vi "FdxCmdRxSAPReadCvi.vi"(8 "error in":errorcluster, 9 "SapReadIn":cluster{"UdpHandle":u32, "MsgCount":u32}, 11 "InstrumentHandle_port":u32) -> (0 "error out":errorcluster, 1 "SapReadOut":cluster{"MsgRead":u32, "ReadBuffer":u8[]}, 3 "InstrumentHandle_port":u32)   [LabVIEW 2020, in "AIM664LV.lvlib"]
doc: "This function reads data from an SAP Connectionless port."
uses:
  AIM664LV.lvlib
  AFDX_LibraryAdmin/FdxGlobalDllPath.vi
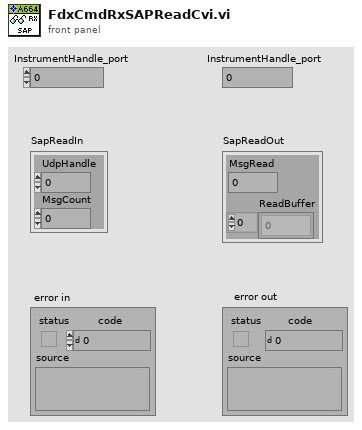
[diagram p1: front panel]
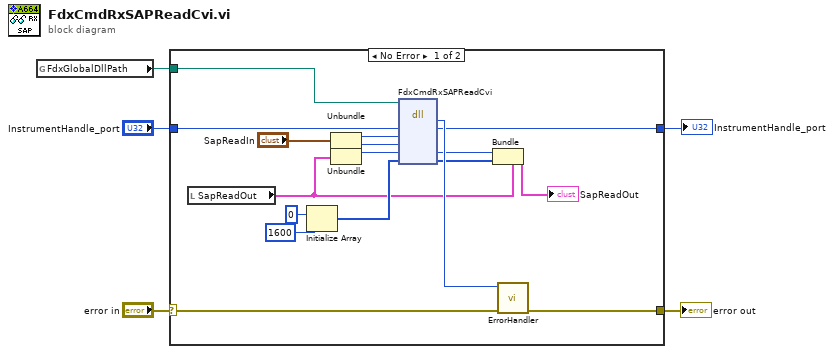
[diagram p0: block diagram]
diagram:
  n1 = global read "FdxGlobalDllPath.vi" "FdxGlobalDllPath"() -> (w3:path)
  n2 = case shown="No Error" "error in" {
    selector: "error in" -> [w21 w24]
    tunnel: [w22 w24] -> w5
    tunnel: w3 -> [w8 _]
    tunnel: "InstrumentHandle_port" -> [w7 w23]
    tunnel: [w6 w23] -> w1
    frame No Error {
      n3 = local read "SapReadOut"() -> (w10:cluster{"MsgRead":u32, "ReadBuffer":u8[]})
      n4 = Initialize Array(u8 0 ("element"), 1600 ("dimension size")) -> (w13:u8[])
      n5 = Unbundle("SapReadIn") -> ("UdpHandle"=w18:u32, "MsgCount"=w17:u32)
      n6 = Unbundle(w10) -> ("MsgRead"=w9:u32)  [unwired: 1 out]
      n7 = dll-call lib="aim_fdx.19.dll" fn="FdxCmdRxSAPReadCvi"(path in=w8, "InstrumentHandle"=w7, "UdpHandle"=w18, "MsgCount"=w17, "MsgRead"=w9, "ReadBuffer"=w13) -> ("status"=w20:i32, "InstrumentHandle"=w6:u32, "MsgRead"=w16:u32, "ReadBuffer"=w12:u8[])  [unwired: 4 in, 2 out]
      n8 = Bundle(cluster=w10, "MsgRead"=w16, "ReadBuffer"=w12) -> (→"SapReadOut":cluster{"MsgRead":u32, "ReadBuffer":u8[]})
      n9 = call "ErrorHandler.vi"("error in"=w21, "AIM Error"=w20) -> ("error out"=w22:errorcluster)  [unwired: 9 in]
    }
    frame Error {
    }
  }
  "error out" <- w5
  "InstrumentHandle_port" <- w1
